vi "Caveat 2.vi"() -> ()   [LabVIEW 2025]
panel:
  out "Loop Iterations":i32
  out "Msg Written Only at Startup":string
  out "Same Msg Written Periodically":string
  # "Caveat #2 UI Only Updates when Remote Panel Connection Active (Must Explicitly Refresh by Writing to Each Indicator)"
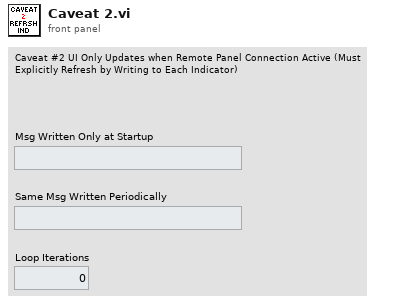
[diagram p1: front panel]
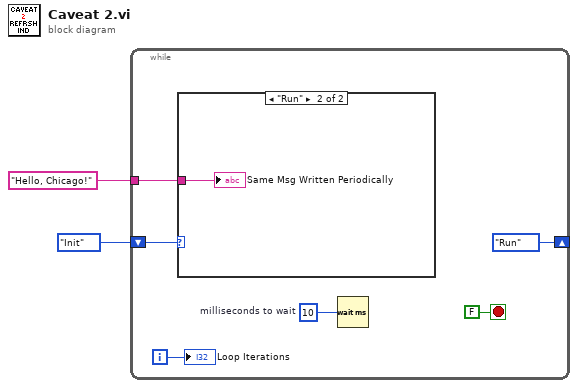
[diagram p0: block diagram]
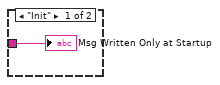
[diagram p2: hidden frame]
diagram:
  n1 = while {
    shift-right: [enum16{"Init", "Run"}."Run"] -> _
    shift-left: enum16{"Init", "Run"}."Init" -> [w6]
    tunnel: "Hello, Chicago!" ("Msg Written Only at Startup") -> [w5]
    i -> [w3]
    stop <- FALSE stop-if-true
    w7 = u32 10  # milliseconds to wait
    n2 = case shown="\"Run\"" w6 {
      tunnel: w5 -> [w9 w10]
      frame "Init" {
        "Msg Written Only at Startup" <- w9
      }
      frame "Run" {
        "Same Msg Written Periodically" <- w10
      }
    }
    n3 = Wait (ms)(milliseconds to wait=w7) -> ()  [unwired: 1 out]
    "Loop Iterations" <- w3
  }
